vi "ini_read_int32s_multi.vi"(7 "section":string, 8 "error in":errorcluster, 9 "defaults":i32[](array[numeric]), 10 "keys (multiline string)":string, 11 "refnum in":T1) -> (0 "error out":errorcluster, 1 "int32s":i32[](array[numeric]), 2 "found?":bool[](array[boolean]), 3 "refnum out":T1)   [LabVIEW 2013]
uses:
  <vilib>/Utility/config.llb/Config Data RefNum.ctl
  <vilib>/Utility/config.llb/NI_LVConfig.lvlib
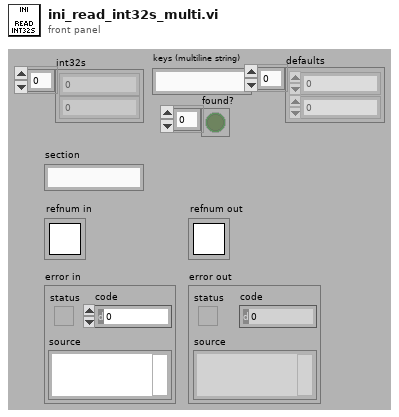
[diagram p1: front panel]
types:
  T1 = typedef "NI_LVConfig.lvlib/Config Data RefNum.ctl" = refnum<k1>
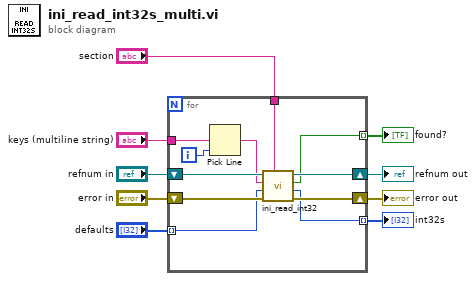
[diagram p0: block diagram]
diagram:
  n1 = for {
    tunnel: "section" -> [w14]
    tunnel: "keys (multiline string)" -> [w20]
    shift-right: [w16] -> w6
    shift-left: "refnum in" -> [w17]
    shift-right: [w15] -> w8
    shift-left: "error in" -> [w18]
    tunnel: "defaults" -> [w12] mode=indexing
    tunnel: [w11] -> w2 mode=indexing
    tunnel: [w10] -> w1 mode=indexing
    i -> [w19]
    n2 = Pick Line(multi-line string=w20, line index=w19) -> (output string=w13:string)  [unwired: 1 in]
    n3 = call "ini_read_int32.vi"("section"=w14, "error in"=w18, "default value"=w12, "key"=w13, "refnum in"=w17) -> ("error out"=w15:errorcluster, "value"=w10:i32, "found?"=w11:bool, "refnum out"=w16:T1)  [unwired: 3 in]
  }
  "error out" <- w8
  "refnum out" <- w6
  "int32s" <- w1
  "found?" <- w2
